vi "session_set_instrument_options.vi"(7 "Item Parsing":T1, 8 "error in":errorcluster caption="error in (no error)", 9 "Options string":string, 11 "VISA resource name":refnum<visa-resource-name>) -> (0 "error out":errorcluster, 1 "Options count":i32, 2 "Options to Session Data":string[](array[string]), 3 "VISA resource name out":refnum<visa-resource-name>)   [LabVIEW 2020, in "Rohde&Schwarz RTx Oscilloscopes.lvlib" / "rsidr_core.lvlib"]
uses:
  rsidr_core.lvlib
  type_Options_Item_Parsing.ctl
  Match Regular Expression.xnode
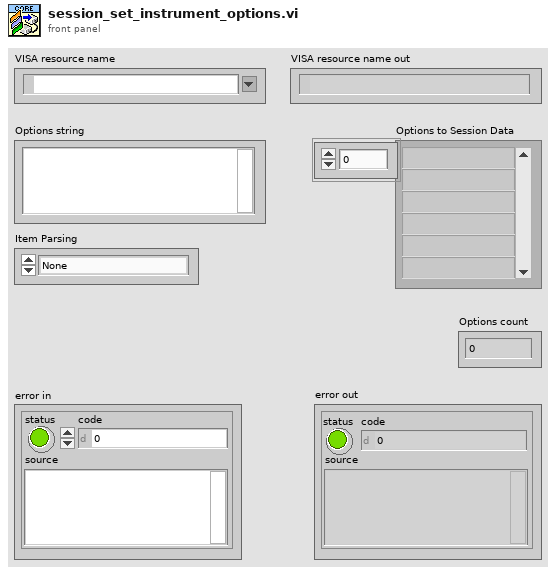
[diagram p1: front panel]
types:
  T1 = typedef "Rohde&Schwarz RTx Oscilloscopes.lvlib/rsidr_core.lvlib/type_Options_Item_Parsing.ctl" = enum16{"None", "Keep parts after dash", "Keep parts before dash", "Automatic"}
  T2 = typedef "Rohde&Schwarz RTx Oscilloscopes.lvlib/rsidr_core.lvlib/type_Session_Data.ctl" = cluster{"IDN string":string, "Instrument FW":string, "Instr type":string, "Instr type for err. msg.":string, "Installed Options":string[], "Ignore Error Messages":string, "Logging params":variant, "OPC Timeout":i32, "VISA Timeout":i32, "STB Poll VISA Timeout":i32, "Additional Flags":i32, "Wait Before Read":i32, "Wait Before Write":i32, "Option String Flags":i32, "IO Segment Size":i64, "VISA Access Mode":T3, "Interface Type":T4, "OPC Wait Mode":T5, "Bin Float Number  Format":T6, "Bin Integer Number Format":T7, "Simulate":bool, "VXIcapable":bool, "Duplicate Session":bool, "Add LF to Write":bool, "Logging":bool, "Fast Sweep":bool, "Query Instrument Status":bool, "Check Range":bool, "Check Options":bool, "OPC-sync Attr Writes":bool, "OPC-sync Attr Queries":bool}
  T3 = typedef "Rohde&Schwarz RTx Oscilloscopes.lvlib/rsidr_core.lvlib/type_VisaAccessMode.ctl" = u16
  T4 = typedef "Rohde&Schwarz RTx Oscilloscopes.lvlib/rsidr_core.lvlib/type_InterfaceType.ctl" = enum16{"Unknown", "GPIB", "VXI", "GPIB_VXI", "ASRL", "PXI", "TCPIP", "USB", "SOCKET"}
  T5 = typedef "Rohde&Schwarz RTx Oscilloscopes.lvlib/rsidr_core.lvlib/type_OPC_Wait_Mode.ctl" = enum16{"STBpolling", "STBpollingSlow", "STBpollingSuperSlow", "ServiceRequest", "OPCquery"}
  T6 = typedef "Rohde&Schwarz RTx Oscilloscopes.lvlib/rsidr_core.lvlib/type_Binary_Float_Number_Format.ctl" = enum16{"Float_4_Bytes_Swapped", "Float_4_Bytes", "Double_8_Bytes_Swapped", "Double_8_Bytes"}
  T7 = typedef "Rohde&Schwarz RTx Oscilloscopes.lvlib/rsidr_core.lvlib/type_Binary_Integer_Number_Format.ctl" = enum16{"Int32_4_Bytes_Swapped", "Int32_4 Bytes", "Int16_2_Bytes_Swapped", "Int16_2_Bytes"}
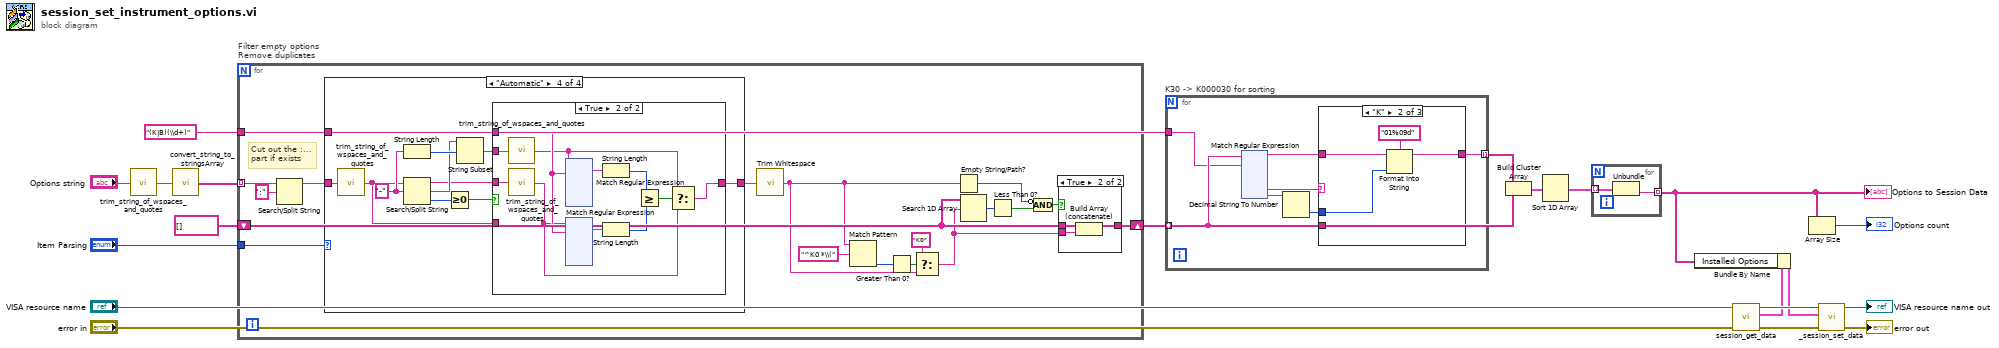
[diagram p0: block diagram]
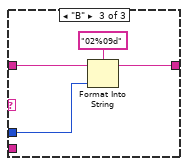
[diagram p3: hidden frame]
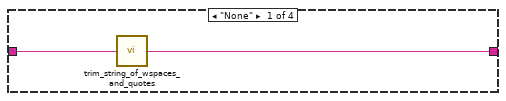
[diagram p4: hidden frame]
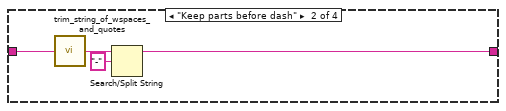
[diagram p5: hidden frame]
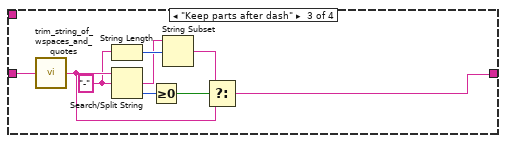
[diagram p6: hidden frame]
diagram:
  w2 = "(K|B)(\\d+)" ("regular expression")
  n1 = call "trim_string_of_wspaces_and_quotes.vi"("String in"="Options string") -> ("String out"=w9:string)  [unwired: 4 in]
  n2 = call "convert_string_to_stringsArray.vi"("String in"=w9) -> ("string array out"=w19:string[])  [unwired: 3 in, 1 out]
  n3 = for "Filter empty options\nRemove duplicates" {
    tunnel: w19 -> [w30] mode=indexing
    shift-right: [w38] -> w1
    shift-left: string[] [] -> [w37]
    tunnel: "Item Parsing" -> [w32]
    tunnel: w2 -> [w27]
    # "Cut out the :...\npart if exists"
    n4 = Search/Split String(string=w30, search string/char (-)=":") -> (substring before match=w29:string)  [unwired: 1 in, 2 out]
    n5 = case shown="\"Automatic\"" w32 {
      tunnel: [w39 w43 w50 w56] -> w28
      tunnel: w29 -> [w40 w42 w53 w64]
      tunnel: w27 -> [_ _ _ w55]
      frame "None" {
        n6 = call "trim_string_of_wspaces_and_quotes.vi"("String in"=w40) -> ("String out"=w39:string)  [unwired: 4 in]
      }
      frame "Keep parts before dash" {
        n7 = call "trim_string_of_wspaces_and_quotes.vi"("String in"=w42) -> ("String out"=w41:string)  [unwired: 4 in]
        n8 = Search/Split String(string=w41, search string/char (-)="-" ("regular expression")) -> (substring before match=w43:string)  [unwired: 1 in, 2 out]
      }
      frame "Keep parts after dash" {
        w46 = "-" ("regular expression")
        n9 = call "trim_string_of_wspaces_and_quotes.vi"("String in"=w53) -> ("String out"=w48:string)  [unwired: 4 in]
        n10 = String Length(string=w46) -> (length=w47:i32)
        n11 = Search/Split String(string=w48, search string/char (-)=w46) -> (match + rest of string=w45:string, offset of match=w52:i32)  [unwired: 1 in, 1 out]
        n12 = Greater Or Equal To 0?(x=w52) -> (x >= 0?=w51:bool)
        n13 = String Subset(string=w45, offset (0)=w47) -> (substring=w49:string)  [unwired: 1 in]
        n14 = Select(t=w49, s=w51, f=w48) -> (s? t:f=w50:string)
      }
      frame "Automatic" {
        w61 = "-" ("regular expression")
        n15 = call "trim_string_of_wspaces_and_quotes.vi"("String in"=w64) -> ("String out"=w58:string)  [unwired: 4 in]
        n16 = String Length(string=w61) -> (length=w62:i32)
        n17 = Search/Split String(string=w58, search string/char (-)=w61) -> (substring before match=w54:string, match + rest of string=w60:string, offset of match=w63:i32)  [unwired: 1 in]
        n18 = Greater Or Equal To 0?(x=w63) -> (x >= 0?=w59:bool)
        n19 = String Subset(string=w60, offset (0)=w62) -> (substring=w57:string)  [unwired: 1 in]
        n20 = case shown="True" w59 {
          tunnel: w58 -> [w65 _]
          tunnel: w57 -> [_ w66]
          tunnel: [w65 w70] -> w56
          tunnel: w55 -> [_ w76]
          tunnel: w54 -> [_ w69]
          frame False {
          }
          frame True {
            n21 = call "trim_string_of_wspaces_and_quotes.vi"("String in"=w66) -> ("String out"=w67:string)  [unwired: 4 in]
            n22 = call "trim_string_of_wspaces_and_quotes.vi"("String in"=w69) -> ("String out"=w68:string)  [unwired: 4 in]
            n23 = xnode ("Match Regular Expression")("input string"=w67, "regular expression"=w76) -> ("whole match"=w75:string)  [unwired: 4 in, 6 out]
            n24 = xnode ("Match Regular Expression")("input string"=w68, "regular expression"=w76) -> ("whole match"=w74:string)  [unwired: 4 in, 6 out]
            n25 = String Length(string=w75) -> (length=w73:i32)
            n26 = String Length(string=w74) -> (length=w72:i32)
            n27 = Greater Or Equal?(x=w73, y=w72) -> (x >= y?=w71:bool)
            n28 = Select(t=w67, s=w71, f=w68) -> (s? t:f=w70:string)
          }
        }
      }
    }
    n29 = call "Trim Whitespace.vi"("string"=w28) -> ("trimmed string"=w23:string)  [unwired: 1 in]
    n30 = Match Pattern(string=w23, regular expression="^K0 *\\(" ("string")) -> (offset past match=w26:i32)  [unwired: 1 in, 3 out]
    n31 = Greater Than 0?(x=w26) -> (x > 0?=w25:bool)
    n32 = Select(t="K0", s=w25, f=w23) -> (s? t:f=w21:string)
    n33 = Empty String/Path?(string/path=w23) -> (empty?=w33:bool)
    n34 = Search 1D Array(1D array=w37, element=w21) -> (index of element=w35:i32)  [unwired: 1 in]
    n35 = Less Than 0?(x=w35) -> (x < 0?=w36:bool)
    n36 = Compound Arithmetic op=AND(invert w33, w36) -> (w34:bool)
    n37 = case shown="True" w34 {
      tunnel: [w305 w306] -> w38
      tunnel: w37 -> [w305 w308]
      tunnel: w21 -> [_ w307]
      frame False {
      }
      frame True {
        n38 = Build Array (concatenate)(w308, w307) -> (w306:string[])
      }
    }
  }
  n39 = for "K30 -> K000030 for sorting" {
    tunnel: w1 -> [w315] mode=indexing
    tunnel: [w314] -> w3 mode=indexing
    tunnel: w2 -> [w309]
    n40 = xnode ("Match Regular Expression")("input string"=w315, "regular expression"=w309) -> ("before match"=w313:string, "submatch 1"=w310:string, "submatch 2"=w312:string)  [unwired: 4 in, 4 out]
    n41 = Decimal String To Number(string=w312) -> (number=w311:i32)  [unwired: 2 in, 1 out]
    n42 = case shown="\"K\"" w310 {
      tunnel: w315 -> [w316 _ _]
      tunnel: [w316 w318 w322] -> w314
      tunnel: w313 -> [_ w319 w323]
      tunnel: w311 -> [_ w317 w321]
      frame Default {
      }
      frame "K" {
        n43 = Format Into String(format string="01%09d", initial string=w319, w317) -> (resulting string=w318:string)  [unwired: 1 in, 1 out]
      }
      frame "B" {
        n44 = Format Into String(format string="02%09d", initial string=w323, w321) -> (resulting string=w322:string)  [unwired: 1 in, 1 out]
      }
    }
  }
  n45 = Build Cluster Array ("Index & Bundle Cluster Array")(w3, w1) -> (w7:cluster{string, string}[])
  n46 = Sort 1D Array(array=w7) -> (sorted array=w6:cluster{string, string}[])
  n47 = for {
    tunnel: w6 -> [w440] mode=indexing
    tunnel: [w439] -> w4 mode=indexing
    n48 = Unbundle(w440) -> (w439:string)  [unwired: 1 out]
  }
  "Options to Session Data" <- w4
  n49 = call "session_get_data.vi"("error in"="error in", "VISA resource name"="VISA resource name") -> ("error out"=w16:errorcluster, "Session User Data out"=w11:T2, "VISA resource name out"=w15:refnum<visa-resource-name>)  [unwired: 6 in, 1 out]
  n50 = Bundle By Name(cluster=w11, "Installed Options"=w4) -> (w12:T2)
  n51 = Array Size(array=w4) -> (size(s)=→"Options count":i32)
  n52 = call "_session_set_data.vi"("error in"=w16, "Session User Data in"=w12, "VISA resource name"=w15) -> ("error out"=→"error out":errorcluster, "VISA resource name out"=→"VISA resource name out":refnum<visa-resource-name>)  [unwired: 7 in]
